vi "Read Current States.vi"(8 "error in (no error)":errorcluster, 11 "ChirpEIS in":refnum<class "ChirpEIS.lvclass">) -> (0 "error out":errorcluster, 2 "Enum":T1=enum."IncreaseVoltage", 3 "ChirpEIS out":refnum<class "ChirpEIS.lvclass">)   [LabVIEW 2014, in "ChirpEIS.lvclass"]
uses:
  ChirpEIS.lvclass
  States.ctl
  ChirpEIS.lvclass/ChirpEIS.ctl
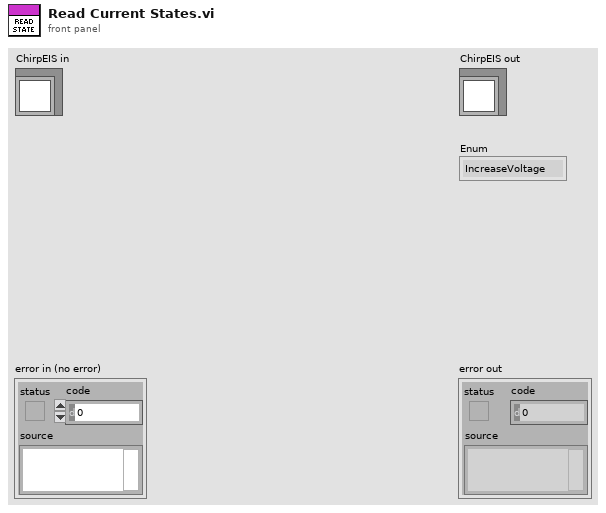
[diagram p1: front panel]
types:
  T1 = typedef "States.ctl" = enum16{"AddDuration", "AddFreq", "CreateNewFile", "Wait", "IncreaseVoltage", "DFT", "ChirpMeasurement", "Initialize", "Ternimate"}
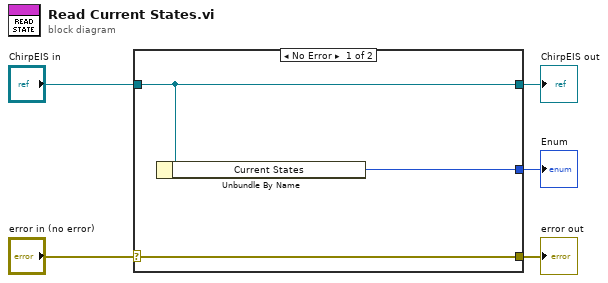
[diagram p0: block diagram]
diagram:
  n1 = case shown="No Error" "error in (no error)" {
    selector: "error in (no error)" -> [w8 w9]
    tunnel: [w8 w9] -> w4
    tunnel: [w7 w10] -> w2
    tunnel: "ChirpEIS in" -> [w7 w10]
    tunnel: [w6 _] -> w1
    frame No Error {
      n2 = Unbundle By Name(w7) -> ("Current States"=w6:T1)
    }
    frame Error {
    }
  }
  "error out" <- w4
  "ChirpEIS out" <- w2
  "Enum" <- w1
